vi "GOMDBTS2048 get TM3015 Coordinates.vi"(8 "error in (no error)":errorcluster, 11 "handle":i32) -> (0 "error out":errorcluster, 2 "function return":i32, 3 "output cluster":T1)   [LabVIEW 2015, in "GOMDBTS2048.lvlib"]
doc: "GOBTS2048DLL int __stdcall GOMDBTS2048_getTM3015Coordinates(int handle, double* TLCoordinates, double* RLCoordinates);"
uses:
  GOMDBTS2048.lvlib
  runtime/GOMDBTS2048.dll
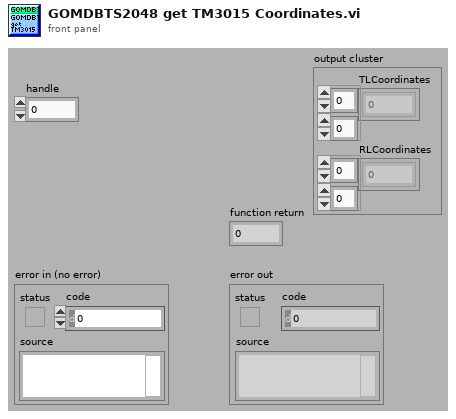
[diagram p1: front panel]
types:
  T1 = cluster{"TLCoordinates":dbl[][], "RLCoordinates":dbl[][]}
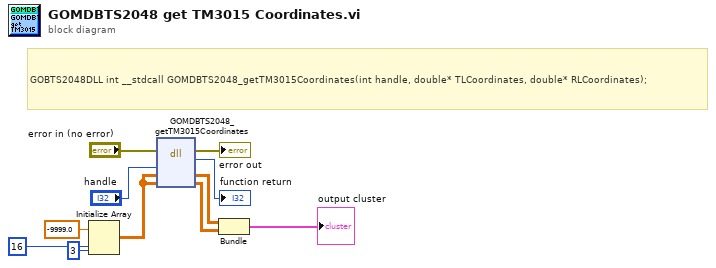
[diagram p0: block diagram]
diagram:
  # "GOBTS2048DLL int __stdcall GOMDBTS2048_getTM3015Coordinates(int handle, double* TLCoordinates, double* RLCoordinates);"
  n1 = Initialize Array(-9999.0 ("element"), 16 ("dimension size"), 3 ("dimension size")) -> (w4:dbl[][])
  n2 = dll-call lib="C:/Users/rkoch/Documents/GO_Library/runtime/GOMDBTS2048.*" fn="GOMDBTS2048_getTM3015Coordinates"(error in="error in (no error)", "handle"="handle", "TLCoordinates"=w4, "RLCoordinates"=w4) -> (error out=→"error out":errorcluster, "return type"=→"function return":i32, "TLCoordinates"=w3:dbl[][], "RLCoordinates"=w2:dbl[][])  [unwired: 3 in, 1 out]
  n3 = Bundle("TLCoordinates"=w3, "RLCoordinates"=w2) -> (→"output cluster":T1)  [unwired: 1 in]
